vi "Write Configuration DVR.vi"(8 "error in (no error)":errorcluster, 10 "framework configuration":T1, 11 "Item Ref in":T17 format="%.0x") -> (0 "error out":errorcluster, 3 "Item Ref out":T17 format="%.0x")   [LabVIEW 2017, in "DSF System Explorer.lvlib"]
uses:
  DSF System Explorer.lvlib
  <vilib>/NI Veristand/Custom Device API/Custom Device Item Ref.ctl
  DSF Core.lvlibp/Typedefs/DSF Engine Framework Configuration.ctl
  DSF Core.lvlibp/Typedefs/DSF Engine Plugin Configuration.ctl
  DSF Core.lvlibp/Typedefs/Core Plugin Configuration.ctl
  DSF Core.lvlibp/Typedefs/DSF Timing Info.ctl
  DSF Core.lvlibp/Typedefs/DSF Settings Info.ctl
  DSF Core.lvlibp/Typedefs/DSF Engine Plugin Thread Configuration.ctl
  DSF Core.lvlibp/Typedefs/Core Thread Configuration.ctl
  DSF Core.lvlibp/Typedefs/DSF Engine Transfer Group Configuration.ctl
  DSF Core.lvlibp/Typedefs/Core Group Configuration.ctl
  DSF Core.lvlibp/Typedefs/DSF Direction.ctl
  DSF Core.lvlibp/Typedefs/DSF Timeout Behavior.ctl
  DSF Core.lvlibp/Typedefs/DSF Engine Transfer Configuration.ctl
  DSF Core.lvlibp/Typedefs/Core Transfer Configuration.ctl
  DSF Core.lvlibp/Typedefs/DSF Engine Channel Configuration.ctl
  DSF Core.lvlibp/Typedefs/Core Channel Configuration.ctl
  DSF Core.lvlibp/Typedefs/DSF Data Type.ctl
  shared data ref.ctl
  <vilib>/NI Veristand/Custom Device API/Get Item Property (U32).vi
  <vilib>/NI Veristand/Custom Device API/Custom Device API.lvlib
  DSF Core.lvlibp
  DSF Core.lvlibp/Classes/Configuration/Base/Channel/Channel Configuration.lvclass
  DSF Core.lvlibp/Classes/Configuration/Base/Transfer/Transfer Configuration.lvclass
  DSF Core.lvlibp/Classes/Configuration/Base/Group/Group Configuration.lvclass
  DSF Core.lvlibp/Classes/Configuration/Base/Thread/Thread Configuration.lvclass
  DSF Core.lvlibp/Classes/Configuration/Base/Plugin/Plugin Configuration.lvclass
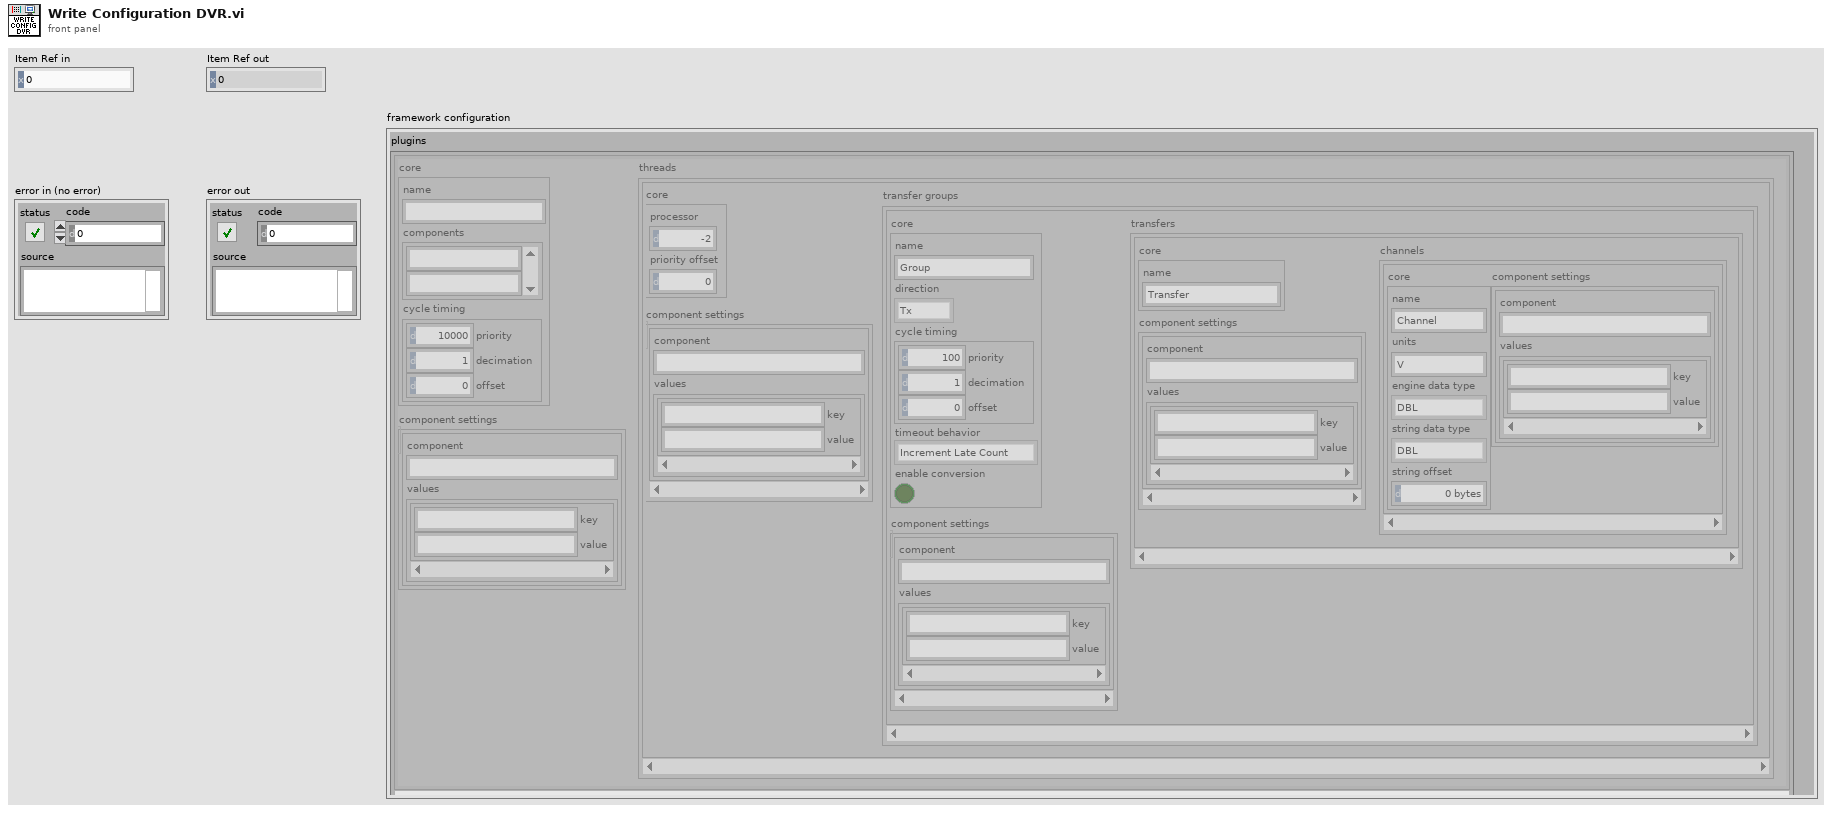
[diagram p1: front panel]
types:
  T1 = typedef "DSF Core.lvlibp/DSF Engine Framework Configuration.ctl" = cluster{"plugins":T2[]}
  T2 = typedef "DSF Core.lvlibp/DSF Engine Plugin Configuration.ctl" = cluster{"core":T3, "component settings":T5[], "threads":T6[]}
  T3 = typedef "DSF Core.lvlibp/Plugin Configuration.lvclass/Core Plugin Configuration.ctl" = cluster{"name":string, "components":string[], "cycle timing":T4}
  T4 = typedef "DSF Core.lvlibp/DSF Timing Info.ctl" = cluster{"priority":u64, "decimation":u64, "offset":u64}
  T5 = typedef "DSF Core.lvlibp/DSF Settings Info.ctl" = cluster{"component":string, "values":cluster{"key":string, "value":string}[]}
  T6 = typedef "DSF Core.lvlibp/DSF Engine Plugin Thread Configuration.ctl" = cluster{"core":T7, "component settings":T5[], "transfer groups":T8[]}
  T7 = typedef "DSF Core.lvlibp/Thread Configuration.lvclass/Core Thread Configuration.ctl" = cluster{"processor":i32, "priority offset":i16}
  T8 = typedef "DSF Core.lvlibp/DSF Engine Transfer Group Configuration.ctl" = cluster{"core":T9, "component settings":T5[], "transfers":T12[]}
  T9 = typedef "DSF Core.lvlibp/Group Configuration.lvclass/Core Group Configuration.ctl" = cluster{"name":string, "direction":T10, "cycle timing":T4, "timeout behavior":T11, "enable conversion":bool}
  T10 = typedef "DSF Core.lvlibp/DSF Direction.ctl" = enum8{"Tx", "Rx"}
  T11 = typedef "DSF Core.lvlibp/DSF Timeout Behavior.ctl" = enum8{"Increment Late Count", "Throw Error"}
  T12 = typedef "DSF Core.lvlibp/DSF Engine Transfer Configuration.ctl" = cluster{"core":T13, "component settings":T5[], "channels":T14[]}
  T13 = typedef "DSF Core.lvlibp/Transfer Configuration.lvclass/Core Transfer Configuration.ctl" = cluster{"name":string}
  T14 = typedef "DSF Core.lvlibp/DSF Engine Channel Configuration.ctl" = cluster{"core":T15, "component settings":T5[]}
  T15 = typedef "DSF Core.lvlibp/Channel Configuration.lvclass/Core Channel Configuration.ctl" = cluster{"name":string, "units":string, "engine data type":T16, "string data type":T16, "string offset":u64}
  T16 = typedef "DSF Core.lvlibp/DSF Data Type.ctl" = enum8{"Bool", "SGL", "DBL", "I8", "I16", "I32", "I64", "U8", "U16", "U32", "U64"}
  T17 = typedef "Custom Device API.lvlib/Custom Device Item Ref.ctl" = u64
  T18 = typedef "DSF System Explorer.lvlib/shared data ref.ctl" = refnum<data-value>
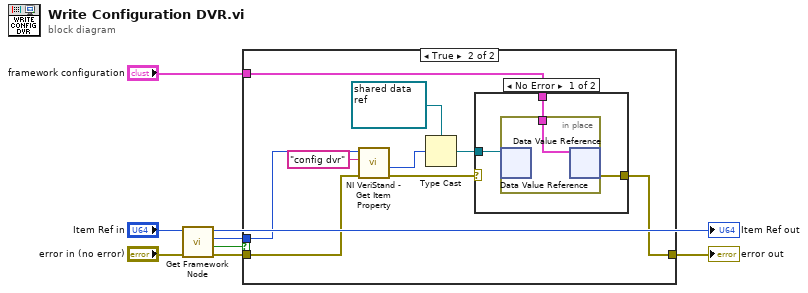
[diagram p0: block diagram]
diagram:
  n1 = call "Get Framework Node.vi"("error in (no error)"="error in (no error)", "Item Ref in"="Item Ref in") -> ("error out"=w6:errorcluster, "found?"=w3:bool, "Framework Ref"=w5:T17, "Item Ref out"=→"Item Ref out":T17)  [unwired: 6 in]
  n2 = case shown="True" w3 {
    tunnel: w6 -> [w9 w13]
    tunnel: w5 -> [_ w12]
    tunnel: [w9 w11] -> w4
    tunnel: "framework configuration" -> [_ w10]
    frame False {
    }
    frame True {
      n3 = call-poly <vilib>:"NI VeriStand - Get Item Property.vi"("error in (no error)"=w13, "Property Name"="config dvr", "Item Ref in"=w12) -> ("error out"=w14:errorcluster, "Value"=w16:u32)  [unwired: 5 in, 2 out]
      n4 = Type Cast(type=T18 refnum ("data value reference"), x=w16) -> (*(type *) &x=w15:T18)
      n5 = case shown="No Error" w14 {
        selector: w14 -> [_ w23]
        tunnel: w15 -> [w21 _]
        tunnel: [w20 w23] -> w11
        tunnel: w10 -> [w19 _]
        frame No Error {
          n6 = in-place {
            in-place-border: w19 -> [w22]
            n7 = in-place-dvr #1(w21) -> ()  [unwired: 2 out]
            n8 = in-place-dvr #1(w22) -> (w20:errorcluster)  [unwired: 1 out]
          }
        }
        frame Error {
        }
      }
    }
  }
  "error out" <- w4
